vi "Brute Force Dark Current Primary Logic Body.vi"(0 "Barcodes in":string[](array[string]), 1 "Stop":bool, 5 "VISA Refnum in":refnum<visa-resource-name>) -> (16 "Bad Tubes":string[](array[string]))   [LabVIEW 2020]
uses:
  Program Files/National Instruments/LabVIEW 2018/instr.lib/CAEN PSM/CAEN PSM.lvlib
panel:
  out "BoardHandle out":T1
  out "error out":errorcluster
  # "INPUTS"
  # "OUTPUTS"
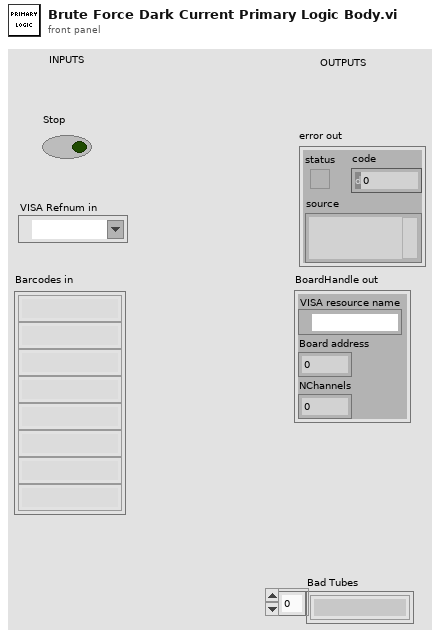
[diagram p1: front panel]
types:
  T1 = cluster{"VISA resource name":refnum<visa-resource-name>, "Board address":u8, "NChannels":u8}
  T2 = typedef "CAEN PSM.lvlib/BoardHandle.ctl" = cluster{"VISA resource name":refnum<visa-resource-name>, "Board address":u8, "NChannels":u8}
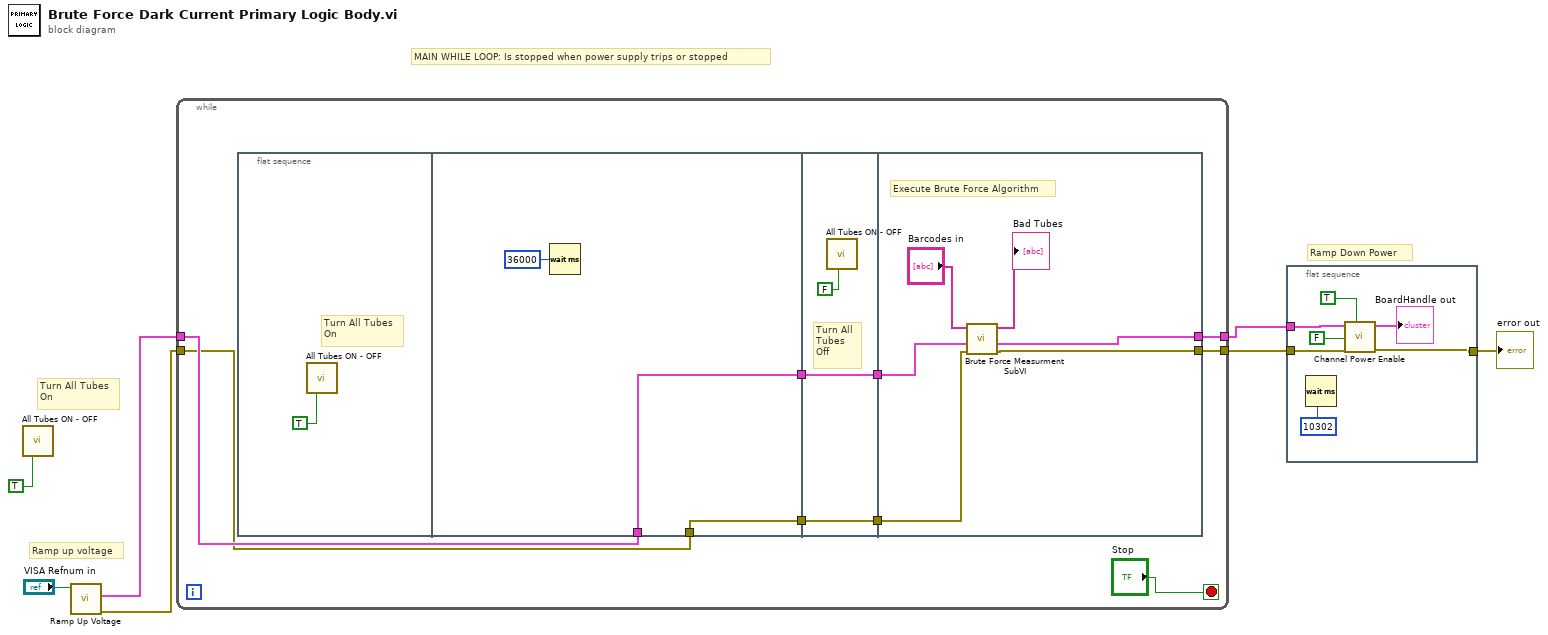
[diagram p0: block diagram]
diagram:
  # "Turn All Tubes \nOn"
  # "Ramp Down Power"
  # "MAIN WHILE LOOP: Is stopped when power supply trips or stopped"
  # "Ramp up voltage"
  n1 = call "All Tubes ON - OFF.vi"("Tubes ON/OFF"=TRUE) -> ()  [unwired: 11 in]
  n2 = call "Ramp Up Voltage.vi"("VISA Refnum in"="VISA Refnum in") -> ("error out"=w2:errorcluster, "BoardHandle out"=w3:T1)  [unwired: 9 in]
  n3 = while {
    tunnel: w3 -> [w10]
    tunnel: [w11] -> w4
    tunnel: w2 -> [w9]
    tunnel: [w12] -> w7
    stop <- "Stop" stop-if-true
    n4 = flat-sequence {
      tunnel: w10 -> [w20]
      tunnel: w9 -> [w19]
      tunnel: [w20] -> w16
      tunnel: [w19] -> w15
      tunnel: [w22] -> w14
      tunnel: w16 -> [w22]
      tunnel: [w21] -> w13
      tunnel: w15 -> [w21]
      tunnel: [w29] -> w12
      tunnel: [w28] -> w11
      tunnel: w14 -> [w25]
      tunnel: w13 -> [w24]
      frame #0 {
        # "Turn All Tubes \nOn"
        n5 = call "All Tubes ON - OFF.vi"("Tubes ON/OFF"=TRUE) -> ()  [unwired: 11 in]
      }
      frame #1 {
        n6 = Wait (ms)(milliseconds to wait=u32 36000) -> ()  [unwired: 1 out]
      }
      frame #2 {
        # "Turn All \nTubes\nOff"
        n7 = call "All Tubes ON - OFF.vi"("Tubes ON/OFF"=FALSE ("Activate: 1\nDeactivate: 0")) -> ()  [unwired: 11 in]
      }
      frame #3 {
        # "Execute Brute Force Algorithm"
        n8 = call "Brute Force Measurment SubVI.vi"("error in (no error)"=w24, "BoardHandle in"=w25, "Barcodes in"="Barcodes in") -> ("error out"=w29:errorcluster, "BoardHandle out"=w28:T1, "Bad Tubes"=→"Bad Tubes":string[])  [unwired: 5 in, 1 out]
      }
    }
  }
  n9 = flat-sequence {
    tunnel: w7 -> [w36]
    tunnel: w4 -> [w35]
    tunnel: [w34] -> w5
    frame #0 {
      n10 = Wait (ms)(milliseconds to wait=u32 10302) -> ()  [unwired: 1 out]
      n11 = call "Channel Power Enable.vi"("All Channels (F)"=TRUE, "error in (no error)"=w36, "Enable (OFF)"=FALSE, "BoardHandle"=w35) -> ("error out"=w34:errorcluster, "BoardHandle out"=→"BoardHandle out":T2)  [unwired: 6 in]
    }
  }
  "error out" <- w5
